vi "纳清pH_所有参数读取.vi"(8 "error in (no error)":errorcluster caption="错误输入（无错误）", 11 "MB session in":refnum<class "MB_Master.lvclass">) -> (0 "error out":errorcluster caption="错误输出", 2 "输出值":T1 {"波特率" items=["4800", "9600", "19200", "38400", "57600", "115200"]}, 3 "MB session out":refnum<class "MB_Master.lvclass">)   [LabVIEW 2016, in "斯坦道多参数.lvlib"]
uses:
  <vilib>/Plasmionique/MB Master/MB_Master/MB_Master.lvclass
  <vilib>/Plasmionique/MB Master/MB Master.lvlib
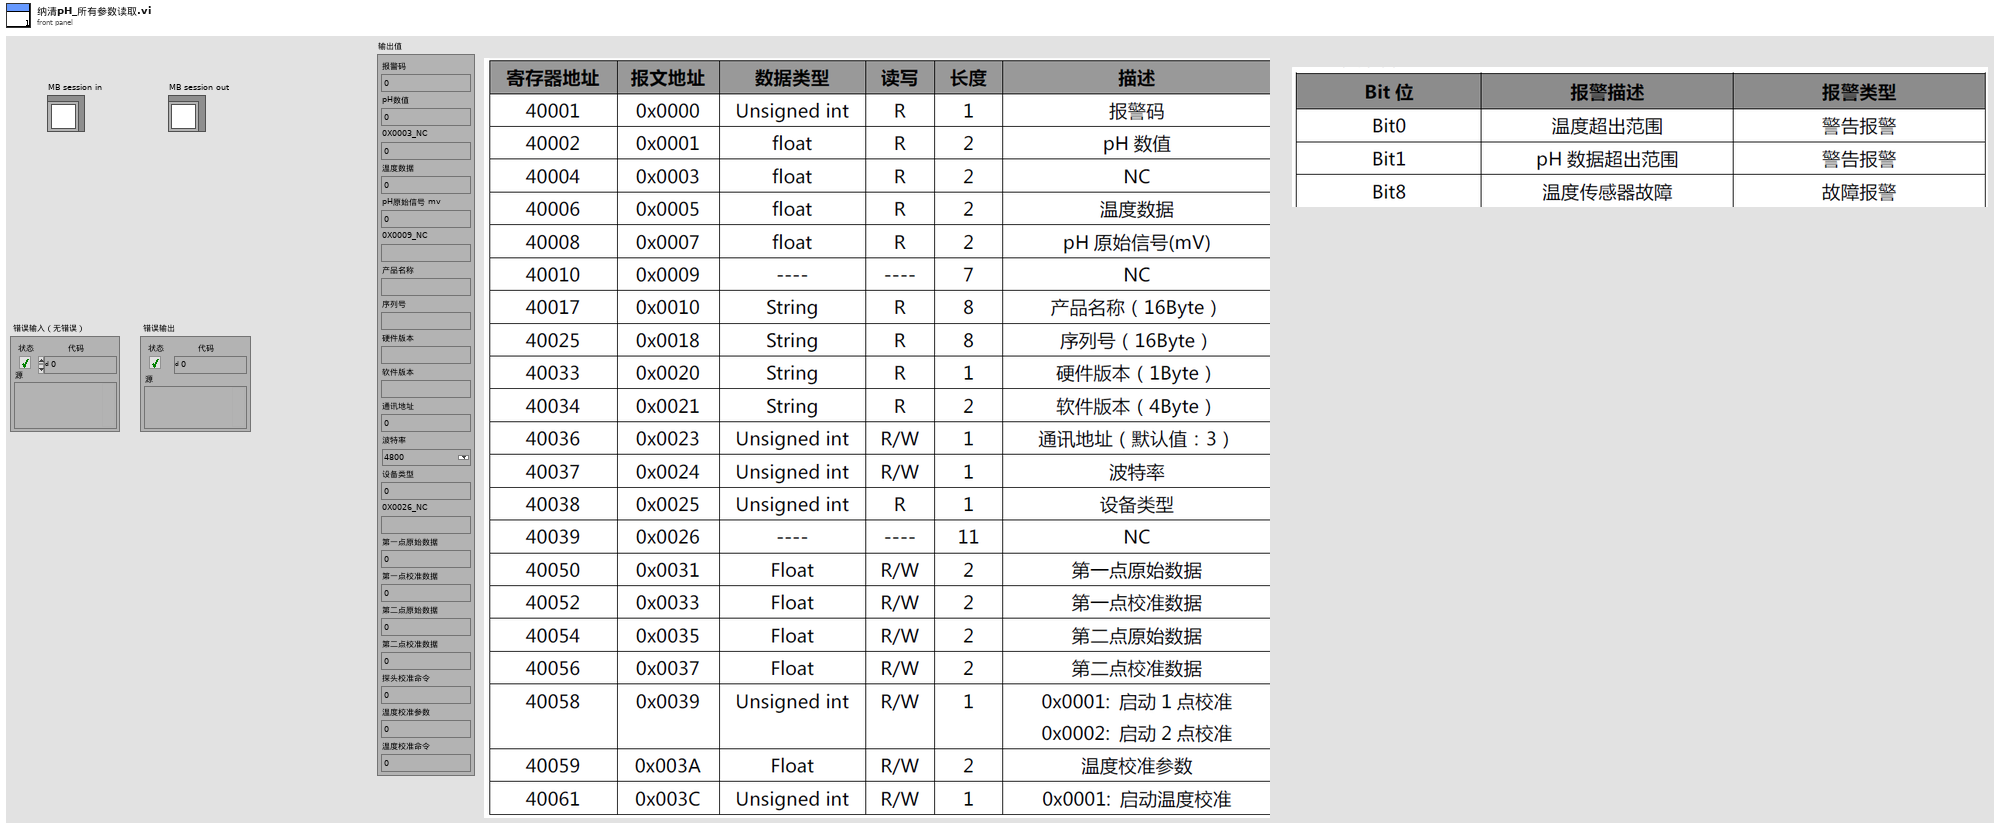
[diagram p1: front panel]
types:
  T1 = cluster{"报警码":u16, "pH数值":sgl, "0X0003_NC":sgl, "温度数据":sgl, "pH原始信号 mv":sgl, "0X0009_NC":string, "产品名称":string, "序列号":string, "硬件版本":string, "软件版本":string, "通讯地址":u16, "波特率":u16, "设备类型":u16, "0X0026_NC":string, "第一点原始数据":sgl, "第一点校准数据":sgl, "第二点原始数据":sgl, "第二点校准数据":sgl, "探头校准命令":u16, "温度校准参数":sgl, "温度校准命令":u16}
  T2 = cluster{"pH":u32, "DO":u32, "Cond":u32, "Turb":u32, "叶绿素a":u32, "藻密度":u32, "ORP":u32, "COD":u32}
  T3 = cluster{u16, "mode":dbl, "数值":sgl, "数值":sgl, "数值":sgl, "类型":string, "类型":string, "类型":string, "类型":string, "类型":string, u16, u16, u16, "类型":string, "数值":sgl, "数值":sgl, "数值":sgl, "数值":sgl, u16, "数值":sgl, u16}
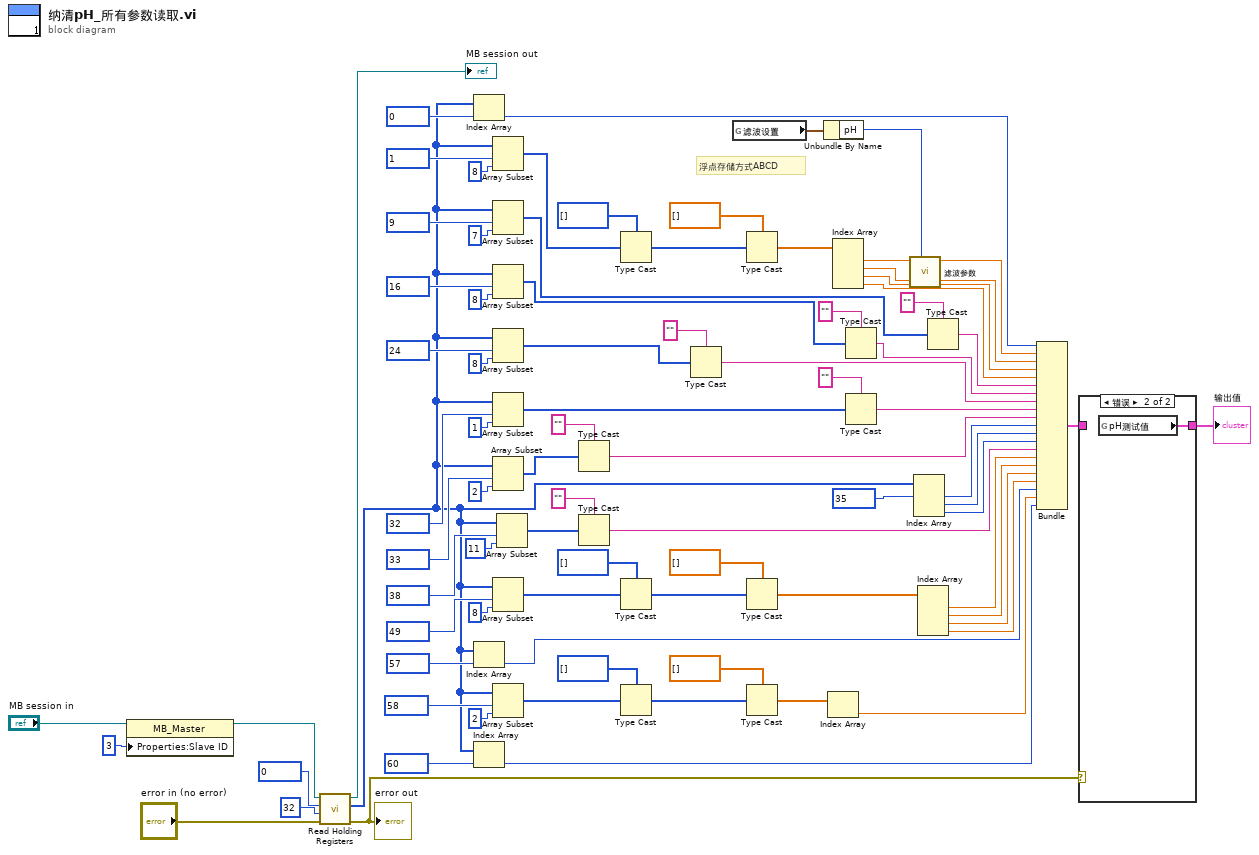
[diagram p0: block diagram]
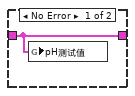
[diagram p2: hidden frame]
diagram:
  # "浮点存储方式ABCD"
  n1 = property class="MB_Master"(reference="MB session in", "Properties:Slave ID"=u8 3 ("Slave ID")) -> (reference out=w74:refnum<class "MB_Master.lvclass">)  [unwired: 1 in, 1 out]
  n2 = call <vilib>:"Read Holding Registers.vi"("error in (no error)"="error in (no error)", "quantity"=u16 32, "starting address"=u16 0, "MB session in"=w74) -> ("error out"=w15:errorcluster, "Registers"=w17:u16[], "MB session out"=→"MB session out":refnum<class "MB_Master.lvclass">)  [unwired: 5 in]
  "error out" <- w15
  n3 = Index Array(array=w17, index=u16 0 ("starting address")) -> (element=w82:u16)
  n4 = Index Array(array=w17, index=u16 57 ("starting address")) -> (element=w20:u16)
  n5 = Index Array(array=w17, index=u16 60 ("starting address")) -> (element=w16:u16)
  n6 = Array Subset(array=w17, index=u16 1 ("starting address"), length=8 ("长度")) -> (w78:u16[])
  n7 = Array Subset(array=w17, index=u16 9 ("starting address"), length=7 ("长度")) -> (w68:u16[])
  n8 = Array Subset(array=w17, index=u16 16 ("starting address"), length=8 ("长度")) -> (w64:u16[])
  n9 = Array Subset(array=w17, index=u16 24 ("starting address"), length=8 ("长度")) -> (w58:u16[])
  n10 = Array Subset(array=w17, index=u16 32 ("starting address"), length=1 ("长度")) -> (w54:u16[])
  n11 = Array Subset(array=w17, index=u16 33 ("starting address"), length=2 ("长度")) -> (w48:u16[])
  n12 = Array Subset(array=w17, index=u16 49 ("starting address"), length=8 ("长度")) -> (w35:u16[])
  n13 = Array Subset(array=w17, index=u16 58 ("starting address"), length=2 ("长度")) -> (w23:u16[])
  n14 = Array Subset(array=w17, index=u16 38 ("starting address"), length=11 ("长度")) -> (w38:u16[])
  n15 = Type Cast(type="" ("类型"), x=w48) -> (*(type *) &x=w46:string)
  n16 = Type Cast(type="" ("类型"), x=w38) -> (*(type *) &x=w37:string)
  n17 = Type Cast(type=u32[] [] ("数组 2"), x=w78) -> (*(type *) &x=w14:u32[])
  n18 = Type Cast(type=u32[] [] ("数组 2"), x=w35) -> (*(type *) &x=w33:u32[])
  n19 = Type Cast(type=u32[] [] ("数组 2"), x=w23) -> (*(type *) &x=w25:u32[])
  n20 = Type Cast(type="" ("类型"), x=w58) -> (*(type *) &x=w56:string)
  n21 = global read "断电保存变量.vi" "滤波设置"() -> (w3:T2)
  n22 = Type Cast(type=sgl[] [] ("数组 2"), x=w14) -> (*(type *) &x=w77:sgl[])
  n23 = Type Cast(type=sgl[] [] ("数组 2"), x=w33) -> (*(type *) &x=w30:sgl[])
  n24 = Type Cast(type=sgl[] [] ("数组 2"), x=w25) -> (*(type *) &x=w28:sgl[])
  n25 = Unbundle By Name(w3) -> ("pH"=w2:u32)
  n26 = Index Array(array=w28) -> (element=w19:sgl)  [unwired: 1 in]
  n27 = Index Array(array=w77) -> (element #1=w5:sgl, element #2=w72:sgl, element #3=w11:sgl, element #4=w10:sgl)  [unwired: 4 in]
  n28 = Type Cast(type="" ("类型"), x=w64) -> (*(type *) &x=w61:string)
  n29 = Type Cast(type="" ("类型"), x=w54) -> (*(type *) &x=w51:string)
  n30 = call "滤波参数.vi"("滤波次数"=w2, "x"=w5) -> ("mode"=w4:dbl)  [unwired: 9 in]
  n31 = Index Array(array=w17, index #1=u16 35 ("starting address")) -> (element #1=w44:u16, element #2=w43:u16, element #3=w42:u16)  [unwired: 2 in]
  n32 = Index Array(array=w30) -> (element #1=w29:sgl, element #2=w9:sgl, element #3=w8:sgl, element #4=w7:sgl)  [unwired: 4 in]
  n33 = Type Cast(type="" ("类型"), x=w68) -> (*(type *) &x=w66:string)
  n34 = Bundle(w82, "mode"=w4, "数值"=w72, "数值"=w11, "数值"=w10, "类型"=w66, "类型"=w61, "类型"=w56, "类型"=w51, "类型"=w46, w44, w43, w42, "类型"=w37, "数值"=w29, "数值"=w9, "数值"=w8, "数值"=w7, w20, "数值"=w19, w16) -> (w6:T3)  [unwired: 1 in]
  n35 = case shown="错误" w15 {
    tunnel: w6 -> [w85 _]
    tunnel: [w85 w86] -> w1
    frame No Error {
      n36 = global write "纳清过程全局变量.vi" "pH测试值"(w85) -> ()
    }
    frame Error {
      n37 = global read "纳清过程全局变量.vi" "pH测试值"() -> (w86:T1)
    }
  }
  "输出值" <- w1
